vi "VectorCased.vi"(8 "DatafileLocation":path, 11 "XYUVArray":dbl[][](array[numeric])=[[-138.0, 28.0, -5.0, -3.0], [-92.0, 28.0, -10.0, -5.5], [-46.0, 28.0, -5.0, -10.5], [0.0, 28.0, -9.0, 3.5], [46.0, 28.0, -22.0, 1.0], [92.0, 28.0, -24.5, -9.0], [138.0, 28.0, -16.0, -23.0], [-138.0, 60.0, -6.0, -2.0], [-92.0, 60.0, -7.0, -12.0], [-46.0, 60.0, -6.0, -11.0], [0.0, 60.0, -9.0, 3.0], [46.0, 60.0, -5.5, 6.0], [92.0, 60.0, -10.0, -7.5], [138.0, 60.0, -17.0, -22.0], [-138.0, 92.0, 0.5, 2.0], [-92.0, 92.0, -1.5, -15.0], [-46.0, 92.0, -1.5, -10.5], [0.0, 92.0, 1.0, -1.5], [46.0, 92.0, 1.0, 3.0], [92.0, 92.0, -2.5, -7.5], [138.0, 92.0, -5.0, -17.0], [-138.0, 124.0, 18.5, 15.0], [-92.0, 124.0, 10.5, -2.5], [-46.0, 124.0, 6.5, -2.0], [0.0, 124.0, 7.5, 5.0], [46.0, 124.0, 9.5, 12.5], [92.0, 124.0, 14.0, 8.5], [138.0, 124.0, 6.5, -4.0], [-138.0, 156.0, 13.5, 14.5], [-92.0, 156.0, 19.5, 4.0], [-46.0, 156.0, 12.5, -1.0], [0.0, 156.0, 10.5, 3.5], [46.0, 156.0, 14.0, 11.0], [92.0, 156.0, 17.5, 10.5], [138.0, 156.0, 12.0, -4.5], [-138.0, 188.0, 9.0, 16.5], [-92.0, 188.0, 10.0, 8.0], [-46.0, 188.0, 14.0, 4.0], [0.0, 188.0, 15.5, 8.0], [46.0, 188.0, 14.5, 11.0], [92.0, 188.0, 21.5, 11.0], [138.0, 188.0, 19.0, 0.5], [-138.0, 214.0, 12.5, 11.5], [-92.0, 214.0, 17.5, 6.0], [-46.0, 214.0, 17.0, 9.5], [0.0, 214.0, 14.5, 10.5], [46.0, 214.0, 19.0, 10.5], [92.0, 214.0, 20.0, 7.0], [138.0, 214.0, 16.5, 7.0]] caption="X                    Y                      U                  V") -> ()   [LabVIEW 2021]
panel:
  out "Display Aspect Ratio":dbl format="%#.2g"
  out "Data Aspect Ratio":dbl format="%#.2g"
  out "Data Y span":dbl
  out "Data X span":dbl
  in  "stop":bool
  in  "Tab Control":enum32{"Data", "Controls", "gnuplot"}(tab)
  in  "VectorScale":dbl(slide)=1.5 min=0.0 step=0.25 scale=0.0..1000.0
  in  "Border":dbl(slide)=0.2 min=0.0 scale=0.0..0.2
  in  "ArrowScale":dbl(slide)=0.3 min=0.0 scale=0.0..0.5
  in  "subfolder":string
  in  "Print Button":bool
  in  "Keep looping":bool=TRUE
  out "VectorPicture":picture
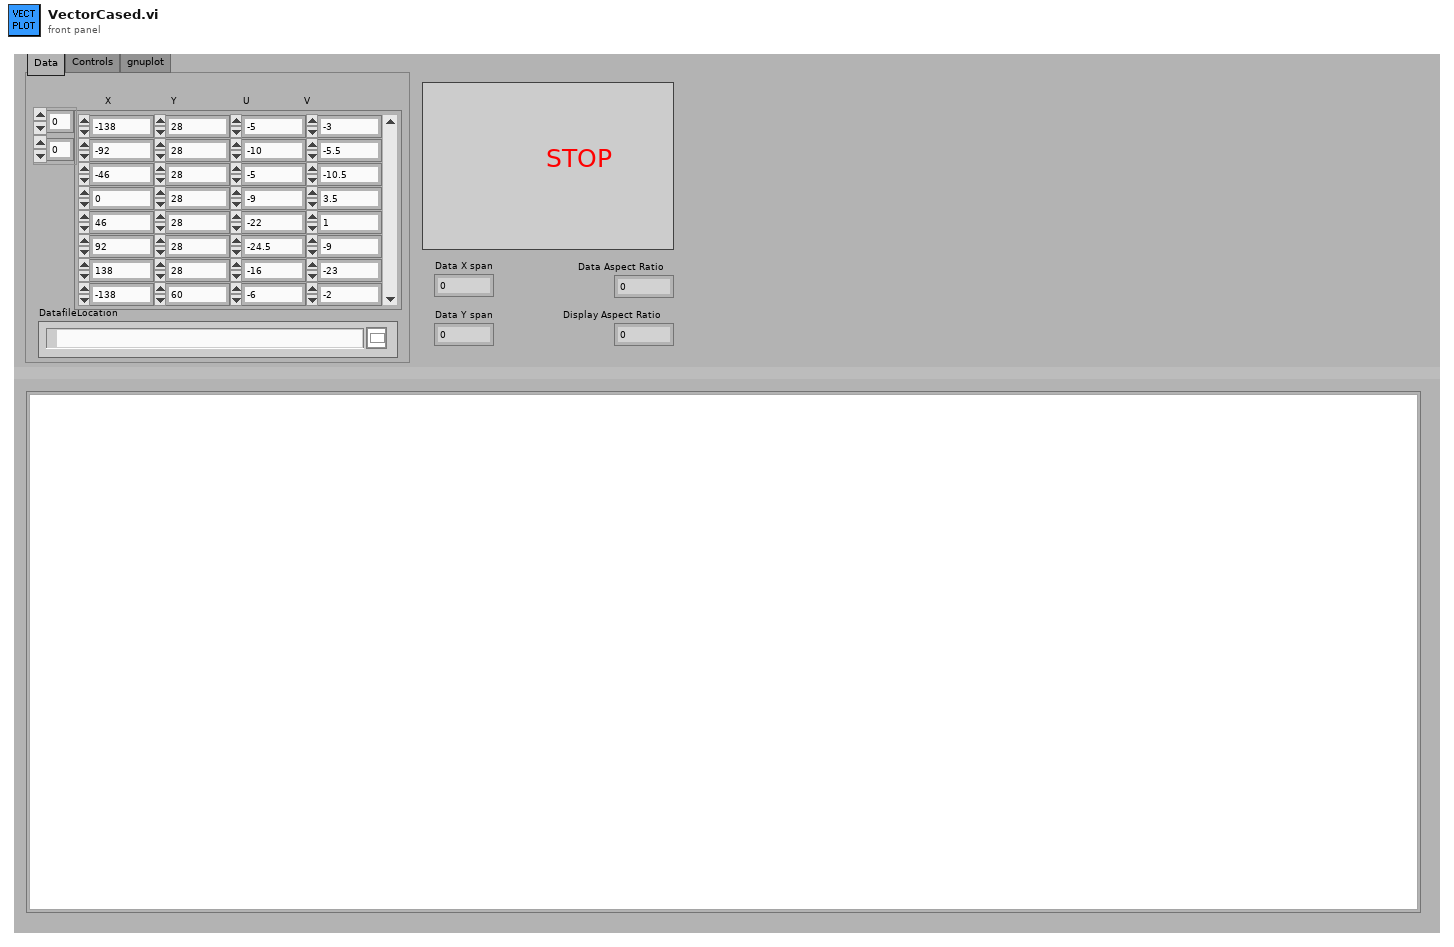
[diagram p1: front panel]
types:
  T1 = typedef "LVBoundsTypeDef.ctl" = cluster{"Width":u32, "Height":u32}
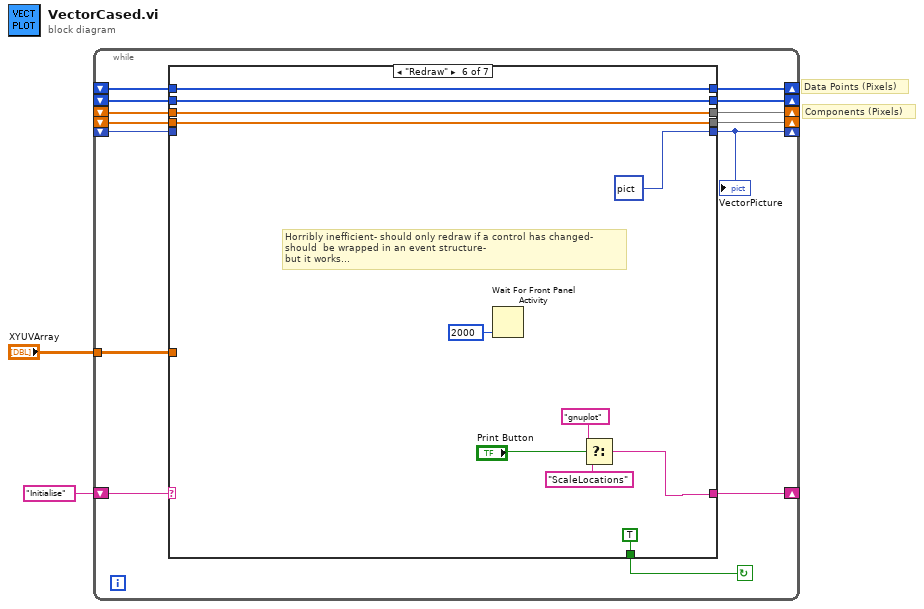
[diagram p0: block diagram]
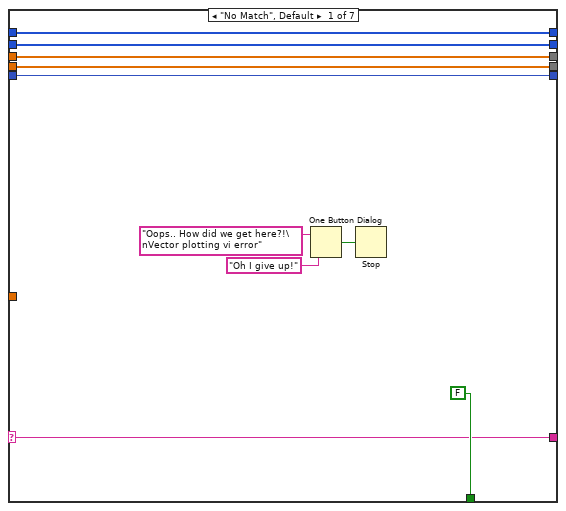
[diagram p2: hidden frame]
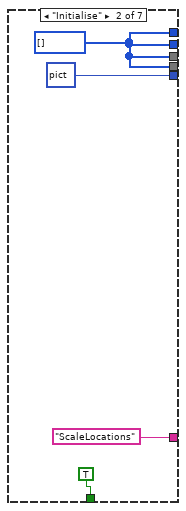
[diagram p3: hidden frame]
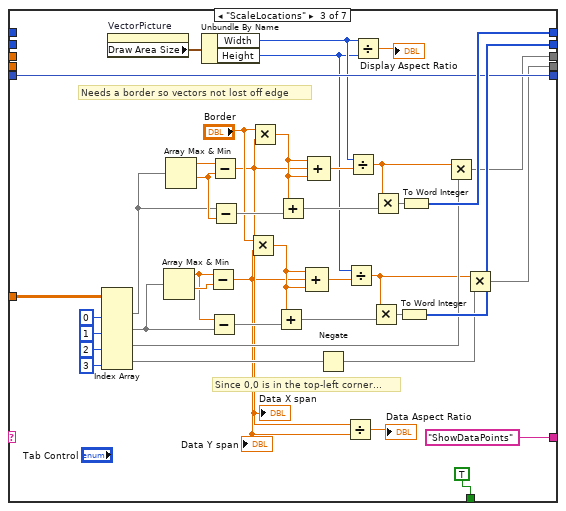
[diagram p4: hidden frame]
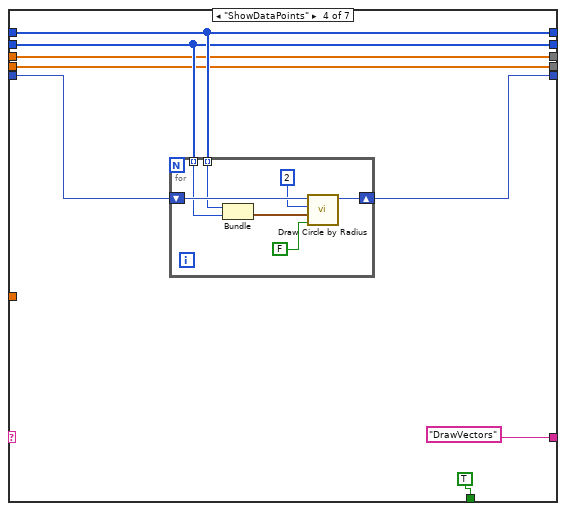
[diagram p5: hidden frame]
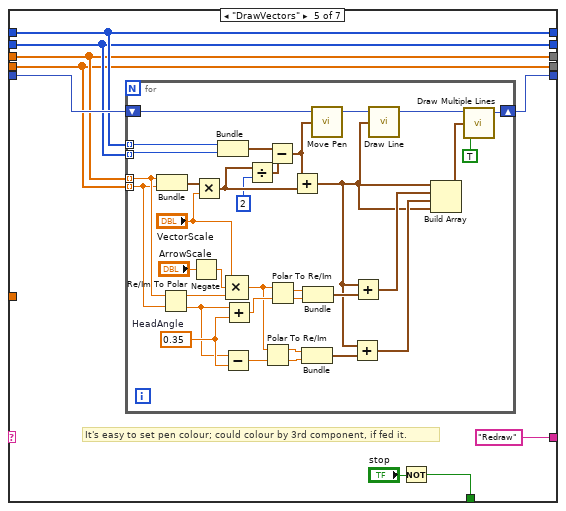
[diagram p6: hidden frame]
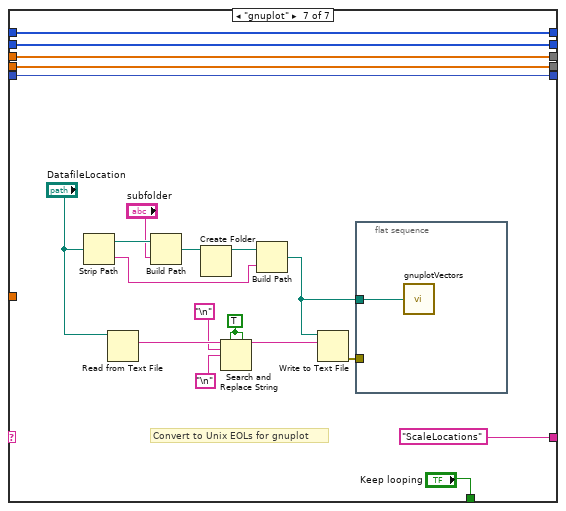
[diagram p7: hidden frame]
diagram:
  # "Components (Pixels)"
  # "Data Points (Pixels)"
  n1 = while {
    shift-right: [w12] -> _
    shift-left: "Initialise" -> [w16]
    shift-right: [w7] -> _
    shift-left: _ -> [w14]
    shift-right: [w11] -> _
    shift-left: _ -> [w9]
    shift-right: [w10] -> _
    shift-left: _ -> [w8]
    shift-right: [w6] -> _
    shift-left: _ -> [w4]
    shift-right: [w5] -> _
    shift-left: _ -> [w3]
    tunnel: "XYUVArray" -> [w13]
    stop <- w15 continue-if-true
    n2 = case shown="\"Redraw\"" w16 {
      selector: w16 -> [w25 _ _ _ _ _ _]
      tunnel: [FALSE TRUE TRUE TRUE w87 TRUE "Keep looping"] -> w15
      tunnel: [w24 picture data[5B] ("new picture") w40 w75 w94 picture data[5B] ("new picture") w156] -> w7
      tunnel: w14 -> [w24 _ w40 w79 w95 _ w156]
      tunnel: w13 -> [_ _ w37 _ _ _ _]
      tunnel: [w25 "ScaleLocations" "ShowDataPoints" "DrawVectors" "Redraw" w134 "ScaleLocations"] -> w12
      tunnel: [w23 w27 w48 w78 w93 w140 w160] -> w11
      tunnel: [w22 w27 w47 w77 w92 w139 w159] -> w10
      tunnel: w9 -> [w23 _ _ w78 w93 w140 w160]
      tunnel: w8 -> [w22 _ _ w77 w92 w139 w159]
      tunnel: [w21 w27 w39 w74 w91 w138 w158] -> w6
      tunnel: [w20 w27 w38 w73 w90 w137 w157] -> w5
      tunnel: w4 -> [w21 _ _ w74 w91 w138 w158]
      tunnel: w3 -> [w20 _ _ w73 w90 w137 w157]
      frame "No Match", Default {
        n3 = One Button Dialog(message="Oops.. How did we get here?!\nVector plotting vi error", button name ("OK")="Oh I give up!") -> (true=w17:bool)
        n4 = Stop(stop? (T)=w17) -> ()
      }
      frame "Initialise" {
        w27 = i16[] []
      }
      frame "ScaleLocations" {
        # "Needs a border so vectors not lost off edge"
        # "Since 0,0 is in the top-left corner..."
        n5 = Index Array(array=w37, index (col) #1=0 ("disabled index (col)"), index (col) #2=1 ("index (col)"), index (col) #3=2 ("index (col)"), index (col) #4=3 ("index (col)")) -> (element #1=w65:dbl[], element #2=w53:dbl[], element #3=w45:dbl[], element #4=w42:dbl[])  [unwired: 4 in]
        n6 = property on="VectorPicture" class="Pict"() -> ("Draw Area Size"=w46:T1)  [unwired: 2 in, 2 out]
        n7 = Array Max & Min(array=w53) -> (max value=w54:dbl, min value=w56:dbl)  [unwired: 2 out]
        n8 = Array Max & Min(array=w65) -> (max value=w71:dbl, min value=w66:dbl)  [unwired: 2 out]
        n9 = Unbundle By Name(w46) -> ("Width"=w32:u32, "Height"=w31:u32)
        n10 = Subtract(x=w54, y=w56) -> (x-y=w35:dbl)
        "Data Y span" <- w35
        n11 = Subtract(x=w54, y=w53) -> (x-y=w57:dbl[])
        n12 = Subtract(x=w71, y=w66) -> (x-y=w36:dbl)
        "Data X span" <- w36
        n13 = Subtract(x=w65, y=w66) -> (x-y=w64:dbl[])
        n14 = Multiply(x="Border", y=w35) -> (x*y=w58:dbl)
        n15 = Multiply(x="Border", y=w36) -> (x*y=w63:dbl)
        n16 = Add(x=w58, y=w57) -> (x+y=w60:dbl[])
        n17 = Add(x=w63, y=w64) -> (x+y=w61:dbl[])
        n18 = Compound Arithmetic op=ADD(w58, w35, w58) -> (w59:dbl)
        n19 = Compound Arithmetic op=ADD(w63, w36, w63) -> (w62:dbl)
        n20 = Negate(x=w42) -> (-x=w41:dbl[])
        n21 = Divide(x=w36, y=w35) -> (x/y=→"Data Aspect Ratio":dbl)
        n22 = Divide(x=w31, y=w59) -> (x/y=w43:dbl)
        n23 = Divide(x=w32, y=w62) -> (x/y=w44:dbl)
        n24 = Divide(x=w32, y=w31) -> (x/y=→"Display Aspect Ratio":dbl)
        n25 = Multiply(x=w43, y=w60) -> (x*y=w49:dbl[])
        n26 = Multiply(x=w44, y=w61) -> (x*y=w50:dbl[])
        n27 = To Word Integer(number=w49) -> (16bit integer=w47:i16[])
        n28 = To Word Integer(number=w50) -> (16bit integer=w48:i16[])
        n29 = Multiply(x=w44, y=w45) -> (x*y=w39:dbl[])
        n30 = Multiply(x=w43, y=w41) -> (x*y=w38:dbl[])
      }
      frame "ShowDataPoints" {
        n31 = for {
          tunnel: w78 -> [w81] mode=indexing
          tunnel: w77 -> [w80] mode=indexing
          shift-right: [w86] -> w75
          shift-left: w79 -> [w84]
          n32 = Bundle(w81, w80) -> (w82:cluster{i16, i16})  [unwired: 1 in]
          n33 = call <vilib>:"Draw Circle by Radius.vi"("fill?(F)"=FALSE, "pixel center"=w82, "radius"=i16 2, "picture"=w84) -> ("new picture"=w86:picture)  [unwired: 7 in]
        }
      }
      frame "DrawVectors" {
        # "It's easy to set pen colour; could colour by 3rd component, if fed it."
        n34 = for {
          tunnel: w91 -> [w119] mode=indexing
          tunnel: w90 -> [w118] mode=indexing
          tunnel: w93 -> [w128] mode=indexing
          tunnel: w92 -> [w127] mode=indexing
          shift-right: [w121] -> w94
          shift-left: w95 -> [w129]
          w107 = 0.35  # HeadAngle
          n35 = Bundle(w119, w118) -> (w122:cluster{dbl, dbl})  [unwired: 1 in]
          n36 = Re/Im To Polar(2:w118, 3:w119) -> (0:w106:dbl, 1:w113:dbl)
          n37 = Negate(x="ArrowScale") -> (-x=w97:dbl)
          n38 = Multiply(x=w122, y="VectorScale") -> (x*y=w126:cluster{dbl, dbl})
          n39 = Bundle(w128, w127) -> (w124:cluster{i16, i16})  [unwired: 1 in]
          n40 = Subtract(x=w106, y=w107) -> (x-y=w103:dbl)
          n41 = Add(x=w106, y=w107) -> (x+y=w114:dbl)
          n42 = Compound Arithmetic op=MULTIPLY("VectorScale", w97, w113) -> (w102:dbl)
          n43 = Divide(x=w126, y=2) -> (x/y=w123:cluster{dbl, dbl})
          n44 = Polar To Re/Im(2:w103, 3:w102) -> (0:w105:dbl, 1:w104:dbl)
          n45 = Subtract(x=w124, y=w123) -> (x-y=w111:cluster{dbl, dbl})
          n46 = Polar To Re/Im(2:w114, 3:w102) -> (0:w116:dbl, 1:w117:dbl)
          n47 = Add(x=w111, y=w126) -> (x+y=w98:cluster{dbl, dbl})
          n48 = Bundle(w104, w105) -> (w101:cluster{dbl, dbl})  [unwired: 1 in]
          n49 = Bundle(w117, w116) -> (w115:cluster{dbl, dbl})  [unwired: 1 in]
          n50 = call <vilib>:"Move Pen.vi"("new position"=w111, "picture"=w129) -> ("new picture"=w109:picture)  [unwired: 3 in]
          n51 = Add(x=w98, y=w101) -> (x+y=w99:cluster{dbl, dbl})
          n52 = Add(x=w98, y=w115) -> (x+y=w100:cluster{dbl, dbl})
          n53 = call <vilib>:"Draw Line.vi"("picture"=w109, "end point"=w98) -> ("new picture"=w108:picture)  [unwired: 7 in]
          n54 = Build Array(w98, w100, w99, w98) -> (w120:cluster{dbl, dbl}[])
          n55 = call <vilib>:"Draw Multiple Lines.vi"("picture"=w108, "line endpoints"=w120, "fill?(F)"=TRUE) -> ("new picture"=w121:picture)  [unwired: 6 in]
        }
        n56 = Not(x="stop") -> (.not. x?=w87:bool)
      }
      frame "Redraw" {
        # "Horribly inefficient- should only redraw if a control has changed-\nshould  be wrapped in an event structure-\nbut it works..."
        n57 = Wait For Front Panel Activity(1:2000 ("timeout ms (-1 never timeout)")) -> ()  [unwired: 2 in, 1 out]
        n58 = Select(t="gnuplot", s="Print Button", f="ScaleLocations") -> (s? t:f=w134:string)
      }
      frame "gnuplot" {
        w151 = TRUE ("multiline? (F)")
        # "Convert to Unix EOLs for gnuplot"
        n59 = Strip Path(path="DatafileLocation") -> (stripped path=w147:path, name=w143:string)
        n60 = Read from Text File(file (use dialog)="DatafileLocation") -> (text=w153:string)  [unwired: 3 in, 3 out]
        n61 = Build Path(base path=w147, name or relative path="subfolder") -> (appended path=w142:path)
        n62 = Create Folder(path (use dialog)=w142) -> (created path=w141:path)  [unwired: 2 in, 2 out]
        n63 = Search and Replace String(replace all?=w151, multiline?=w151, input string=w153, search string="\n", replace string="\n") -> (result string=w149:string)  [unwired: 3 in, 3 out]
        n64 = Build Path(base path=w141, name or relative path=w143) -> (appended path=w144:path)
        n65 = Write to Text File(file (use dialog)=w144, text=w149) -> (error out=w146:errorcluster)  [unwired: 2 in, 2 out]
        n66 = flat-sequence {
          tunnel: w144 -> [w161]
          tunnel: w146 -> [_]
          frame #0 {
            n67 = call "gnuplotVectors.vi"("VectorFileLocation"=w161) -> ()  [unwired: 2 in, 3 out]
          }
        }
      }
    }
    "VectorPicture" <- w7
  }
